vi "Read Files.vi"(8 "error in (no error)":errorcluster, 11 "Tree Data Folder in":refnum<class "Tree Data Folder.lvclass">) -> (0 "error out":errorcluster, 2 "Files":refnum<class "Tree Data File.lvclass">[](array[class]), 3 "Tree Data Folder out":refnum<class "Tree Data Folder.lvclass">)   [LabVIEW 2022 SP3, in "Tree Data Folder.lvclass"]
uses:
  Tree Data Folder.lvclass
  Tree Data File/Tree Data File.lvclass
  Tree Data Folder.lvclass/Tree Data Folder.ctl
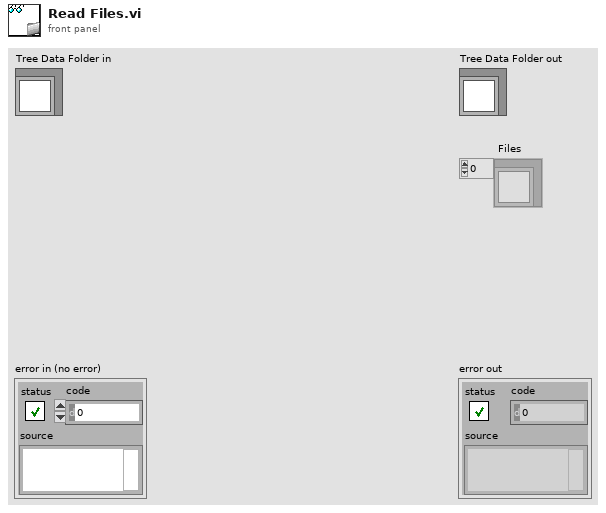
[diagram p1: front panel]
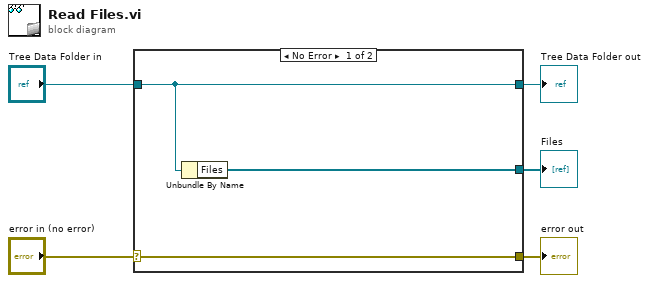
[diagram p0: block diagram]
diagram:
  n1 = case shown="No Error" "error in (no error)" {
    selector: "error in (no error)" -> [w8 w9]
    tunnel: [w8 w9] -> w4
    tunnel: [w7 w10] -> w2
    tunnel: "Tree Data Folder in" -> [w7 w10]
    tunnel: [w6 _] -> w1
    frame No Error {
      n2 = Unbundle By Name(w7) -> ("Files"=w6:refnum<class "Tree Data File.lvclass">[])
    }
    frame Error {
    }
  }
  "error out" <- w4
  "Tree Data Folder out" <- w2
  "Files" <- w1
